vi "Template Get by ixTemplate.vi"(8 "error in (no error)":errorcluster, 10 "ixTemplate (0)":i32, 11 "Connection Refnum":T1) -> (0 "error out":errorcluster, 2 "Template Record":T2, 3 "Connection Refnum":T1, 4 "Data Present":bool)   [LabVIEW 2011]
uses:
  Template Record.ctl
  SI.LIB/ODBC/SQL Controls/Connection Refnum.ctl
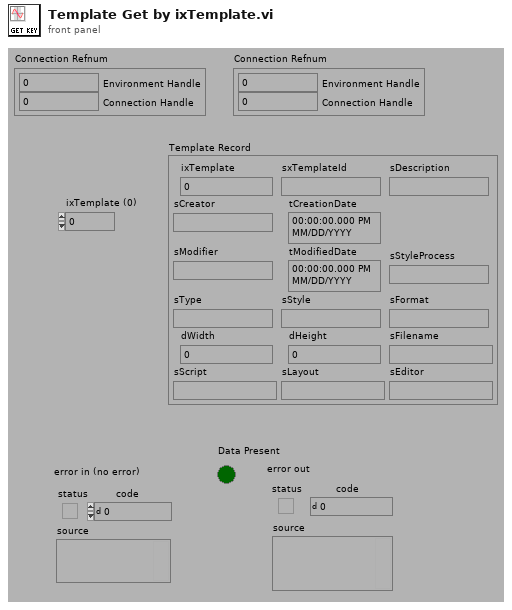
[diagram p1: front panel]
types:
  T1 = typedef "Connection Refnum.ctl" = cluster{"Environment Handle":i32, "Connection Handle":i32}
  T2 = typedef "Template Record.ctl" = cluster{"ixTemplate":i32, "sxTemplateId":string, "sDescription":string, "sCreator":string, "tCreationDate":timestamp, "sModifier":string, "tModifiedDate":timestamp, "sType":string, "sStyle":string, "sFormat":string, "dWidth":dbl, "dHeight":dbl, "sFilename":string, "sScript":string, "sLayout":string, "sEditor":string, "sStyleProcess":string}
  T3 = typedef "Statement Refnum.ctl" = cluster{"Statement Handle":i32, "Parameter Number":u16}
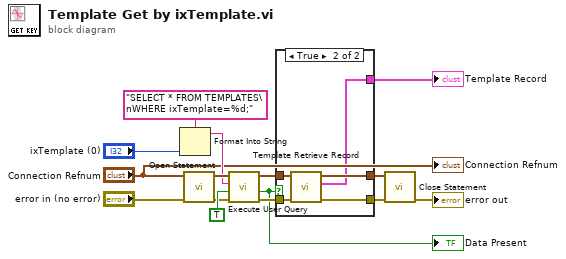
[diagram p0: block diagram]
diagram:
  n1 = Format Into String(format string="SELECT * FROM TEMPLATES\nWHERE ixTemplate=%d;" ("User Query"), "ixTemplate (0)") -> (resulting string=w7:string)  [unwired: 2 in, 1 out]
  n2 = call "Open Statement.vi"("error in (no error)"="error in (no error)", "Connection Refnum"="Connection Refnum") -> ("error out"=w8:errorcluster, "Statement Refnum"=w9:T3)  [unwired: 4 out]
  n3 = call "Execute User Query.vi"("error in (no error)"=w8, "Return Data? (f)"=TRUE, "User Query"=w7, "Statement Refnum"=w9) -> ("error out"=w15:errorcluster, "Data Present?"=w3:bool, "Statement Refnum"=w14:T3)  [unwired: 1 out]
  "Data Present" <- w3
  n4 = case shown="True" w3 {
    tunnel: w15 -> [w16 w21]
    tunnel: w14 -> [w17 w22]
    tunnel: [w16 w19] -> w11
    tunnel: [w17 w20] -> w12
    tunnel: [_ w18] -> w2
    frame False {
    }
    frame True {
      n5 = call "Template Retrieve Record.vi"("error in (no error)"=w21, "Statement Refnum"=w22) -> ("error out"=w19:errorcluster, "Template Record"=w18:T2, "Statement Refnum"=w20:T3)  [unwired: 7 out]
    }
  }
  "Template Record" <- w2
  n6 = call "Close Statement.vi"("error in (no error)"=w11, "Statement Refnum"=w12) -> ("error out"=→"error out":errorcluster)  [unwired: 5 out]
  "Connection Refnum" <- "Connection Refnum"
